vi "Write Last Waveforms.vi"(8 "error in (no error)":errorcluster, 10 "Last Waveforms":map{u8, waveform(dbl)}(c390), 11 "Scope Base in":refnum<class "Scope Base.lvclass">) -> (0 "error out":errorcluster, 3 "Scope Base out":refnum<class "Scope Base.lvclass">)   [LabVIEW 2023, in "Scope.lvlib" / "Scope Base.lvlib" / "Scope Base.lvclass"]
uses:
  Scope Base.lvclass
  Scope Base.lvclass/Scope Base.ctl
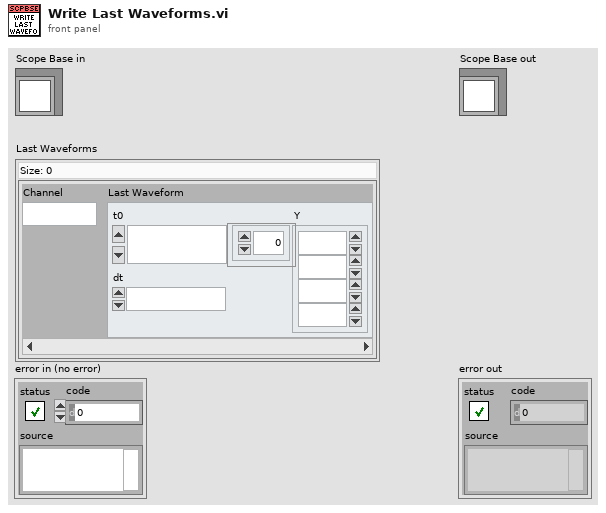
[diagram p1: front panel]
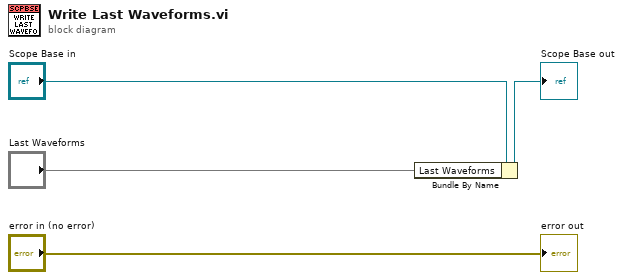
[diagram p0: block diagram]
diagram:
  n1 = Bundle By Name(cluster="Scope Base in", "Last Waveforms"="Last Waveforms") -> (→"Scope Base out":refnum<class "Scope Base.lvclass">)
  "error out" <- "error in (no error)"
